vi "Record Frame Mouse Metadata.vi"(4 "Frame Number":u32, 5 "Right Button Click":bool, 6 "Relative seconds":dbl format="%#_13g", 7 "Left Button Click":bool, 8 "error in":errorcluster, 9 "Cursor Position Y":i32, 10 "Cursor Position X":i32, 11 "Module ID":i32=-1) -> (0 "error out":errorcluster)   [LabVIEW 2026, in "UserEventRecorder.lvlib"]
doc: "_____\nCreated using DQMH Framework: Event Scripter 7.1.2.1547."
uses:
  UserEventRecorder.lvlib
  Record Frame Mouse Metadata Argument--cluster.ctl
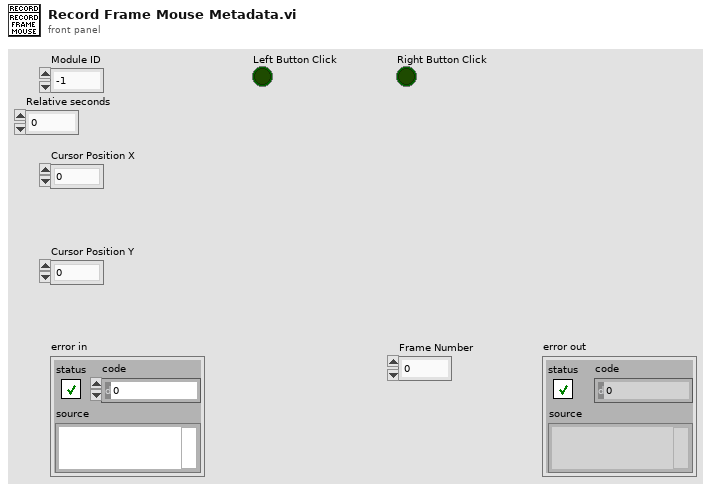
[diagram p1: front panel]
types:
  T1 = typedef "UserEventRecorder.lvlib/Record Frame Mouse Metadata Argument--cluster.ctl" = cluster{"Module ID":i32, "Cursor Position X":i32, "Cursor Position Y":i32, "Left Button Click":bool, "Right Button Click":bool, "Frame Number":u32, "Relative seconds":dbl}
  T2 = typedef "UserEventRecorder.lvlib/Request Events--cluster.ctl" = cluster{"Stop Module":refnum<user-event>, "Show Panel":refnum<user-event>, "Hide Panel":refnum<user-event>, "Show Diagram":refnum<user-event>, "Get Module Execution Status":refnum<user-event>, "Record Frame Mouse Metadata":refnum<user-event>}
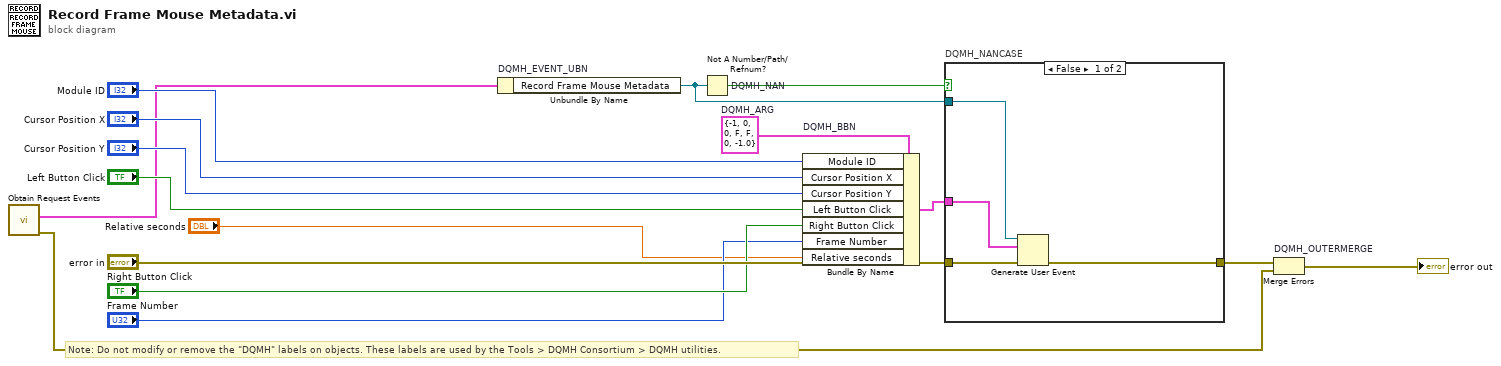
[diagram p0: block diagram]
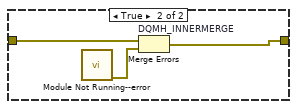
[diagram p2: hidden frame]
diagram:
  w10 = T1 {"Module ID"=-1, "Cursor Position X"=0, "Cursor Position Y"=0, "Left Button Click"=FALSE, "Right Button Click"=FALSE, "Frame Number"=0, "Relative seconds"=-1.0}  # DQMH_ARG
  # "Note: Do not modify or remove the \"DQMH\" labels on objects. These labels are used by the Tools > DQMH Consortium > DQMH utilities."
  n1 = call "Obtain Request Events.vi"() -> ("error out"=w3:errorcluster, "UserEventRecorder Request Events"=w2:T2)  [unwired: 10 in]
  n2 = Unbundle By Name "DQMH_EVENT_UBN"(w2) -> ("Record Frame Mouse Metadata"=w12:refnum<user-event>)
  n3 = Not A Number/Path/Refnum? "DQMH_NAN"(number/path/refnum=w12) -> (NaN/Path/Refnum?=w13:bool)
  n4 = Bundle By Name "DQMH_BBN"(cluster=w10, "Module ID"="Module ID", "Cursor Position X"="Cursor Position X", "Cursor Position Y"="Cursor Position Y", "Left Button Click"="Left Button Click", "Right Button Click"="Right Button Click", "Frame Number"="Frame Number", "Relative seconds"="Relative seconds") -> (w14:T1)
  n5 = case "DQMH_NANCASE" shown="False" w13 {
    tunnel: "error in" -> [w20 w23]
    tunnel: [w19 w22] -> w11
    tunnel: w12 -> [w18 _]
    tunnel: w14 -> [w17 _]
    frame False {
      n6 = Generate User Event(user event=w18, event data cluster=w17, error in=w20) -> (error out=w19:errorcluster)  [unwired: 1 in, 1 out]
    }
    frame True {
      n7 = call "Module Not Running--error.vi"() -> ("error out"=w21:errorcluster)  [unwired: 11 in]
      n8 = Merge Errors "DQMH_INNERMERGE"(w23, w21) -> (w22:errorcluster)
    }
  }
  n9 = Merge Errors "DQMH_OUTERMERGE"(w11, w3) -> (→"error out":errorcluster)
